vi "FilterWheelPan.vi"(8 "error in (no error)":errorcluster caption="entrée d'erreur (pas d'erreur)", 11 "AppliedMotionDrive.lvclass":refnum<class "AppliedMotionDrive.lvclass">) -> (0 "error out":errorcluster caption="sortie d'erreur", 3 "AppliedMotionDrive.lvclass Out":refnum<class "AppliedMotionDrive.lvclass">)   [LabVIEW 2019, in "AppliedMotionDrive.lvclass"]
uses:
  AppliedMotionDrive.lvclass
  C:/Programmes Labview/LabscanV1A/DevicesClass/BaseDevice/BaseDevice.lvclass
  AppliedMotionDrive.lvclass/AppliedMotionDrive.ctl
  BaseDevice/ClassQueueMess.ctl
  BaseDevice/Accessor/GetClassEvent.vi
panel:
  in  "Auto APD":bool
  out "ESP300Mirror":u16=1
  out "ESP300Filters":u16=1
  out "APDsRefs":refnum<vi>[](array[refnum])
  out "LampRefs":refnum<vi>[](array[refnum])
  out "DelayedClosed":bool caption="Confirm"
  out "Delay (hours)":dbl format="%#g"
  out "RéfMenu":refnum<k9>
  in  "White Lamp":bool
  in  "MainProgQEvent":refnum<user-event>
  in  "MainProgQ":refnum<queue>
  out "Offet(Units)":dbl caption="Offset(Units)"
  in  "APDs":bool
  in  "PosDelta(Units)":dbl caption="Pos delta(mm)"
  in  "Con":bool
  in  "TimeoutCnt":u32
  in  "Err":bool
  out "DisAtPos":bool
  out "Acq":bool
  in  "Filter pos(Units)":dbl caption="FiltPos(mm)"
  in  "Home":bool
  in  "En":bool
  in  "Filters":u16(ring) items=["test"]
  out "InstrName":string="Filter Wheel"
  out "Moving":bool
  in  "Stop Move":bool
  in  "Position(Units)":dbl caption="Position(mm)"
  in  "Stop":bool
  out "Init Program":bool
  # "this MUST labeled with class name"
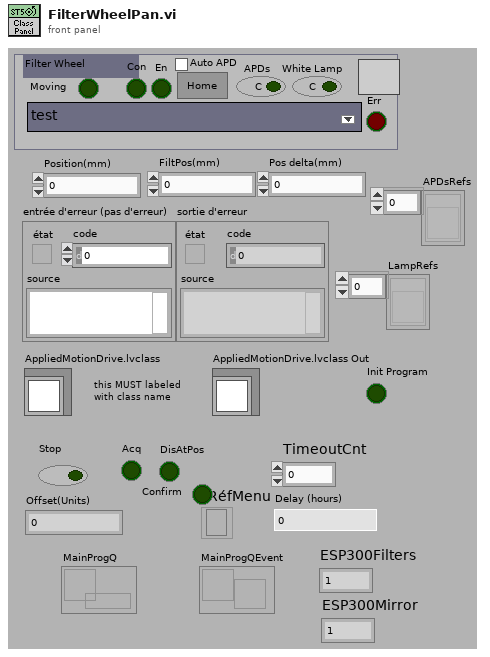
[diagram p1: front panel]
types:
  T1 = cluster{"Enabled":bool, "Sampling":bool, "Fault":bool, "In Position":bool, "Moving":bool, "Jogging":bool, "Stopping":bool, "Wait Input":bool, "Saving":bool, "Alarm":bool, "Homing":bool, "Waiting":bool, "Wait Time":bool, "Wizard":bool, "Checking Enc":bool, "Q mode":bool, "Initializing":bool}
  T2 = cluster{"Vitesse (Tour/s)":dbl, "Accél":dbl, "Décél":dbl, "Accél Max":dbl, "Idle Current (A) ":dbl}
  T3 = cluster{"Vitesse (Tour/s)":dbl, "Accél":dbl, "Décél":dbl}
  T4 = typedef "ClassQueueMess.ctl" = u16
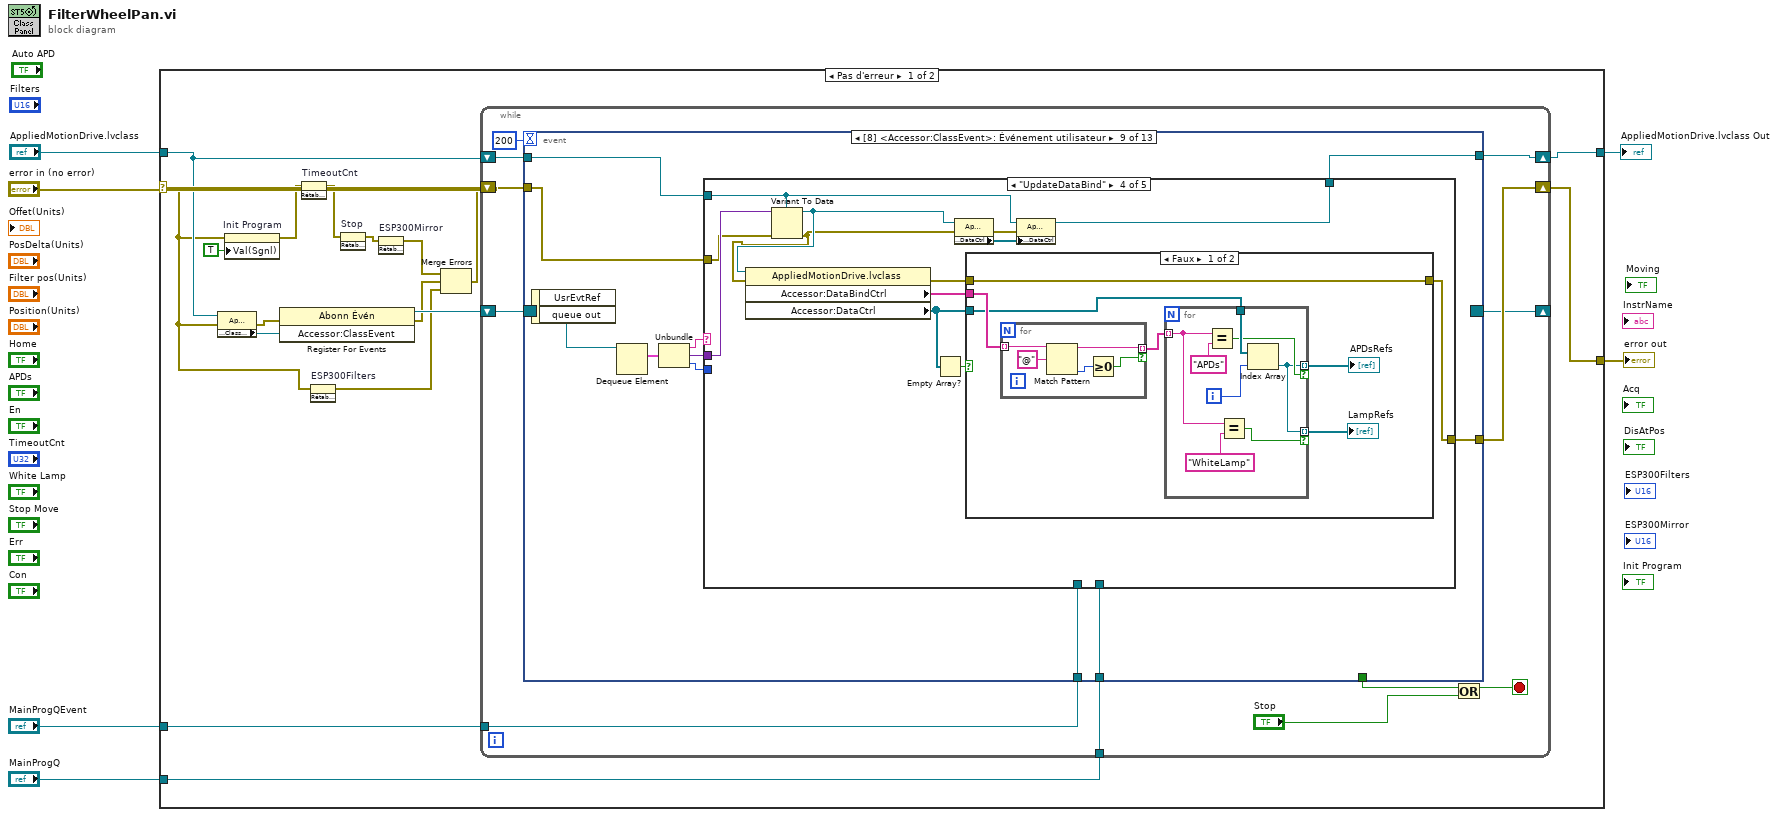
[diagram p0: block diagram]
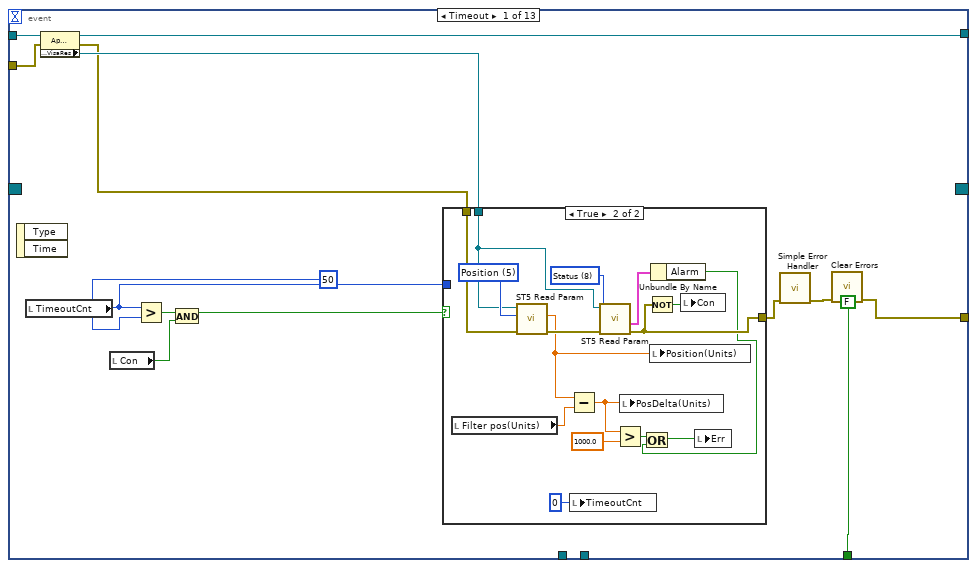
[diagram p2: hidden frame]
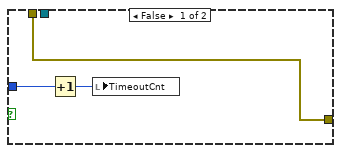
[diagram p3: hidden frame]
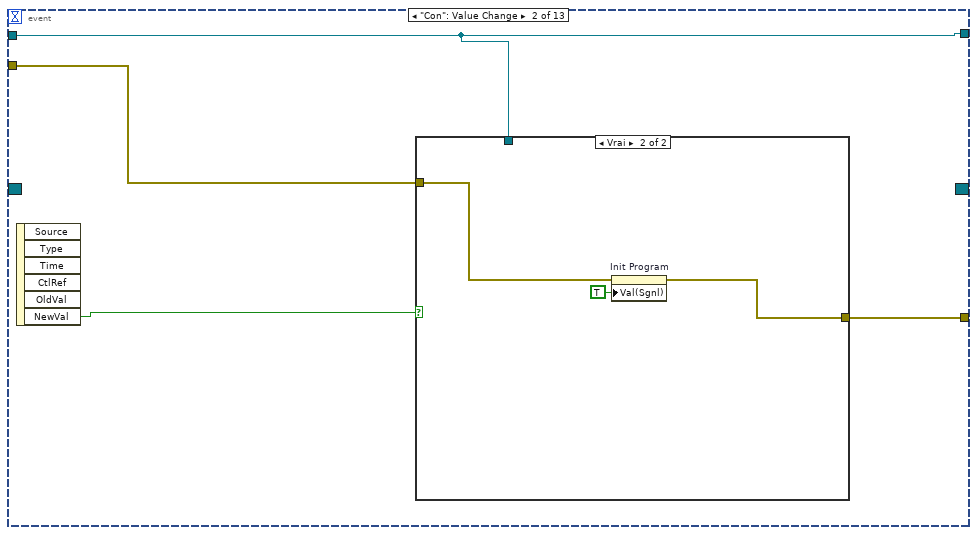
[diagram p4: hidden frame]
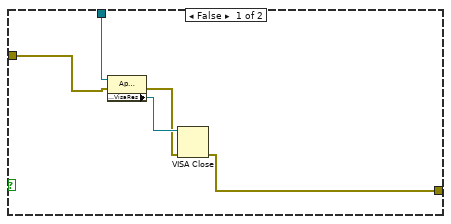
[diagram p5: hidden frame]
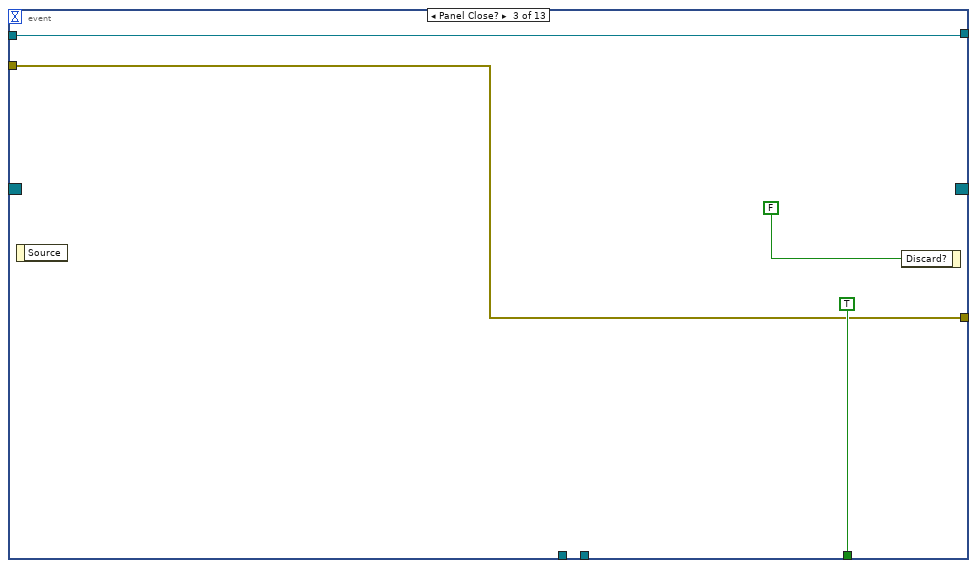
[diagram p6: hidden frame]
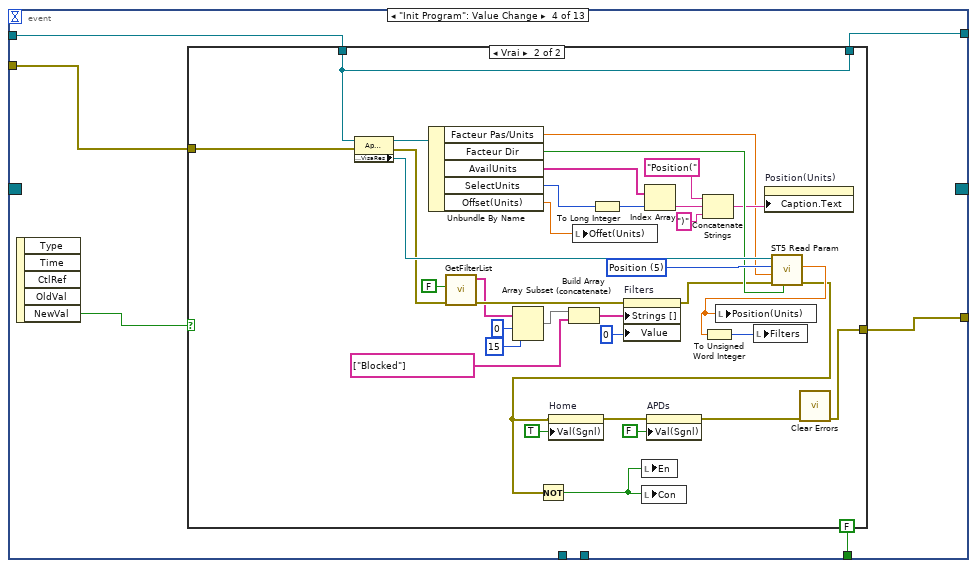
[diagram p7: hidden frame]
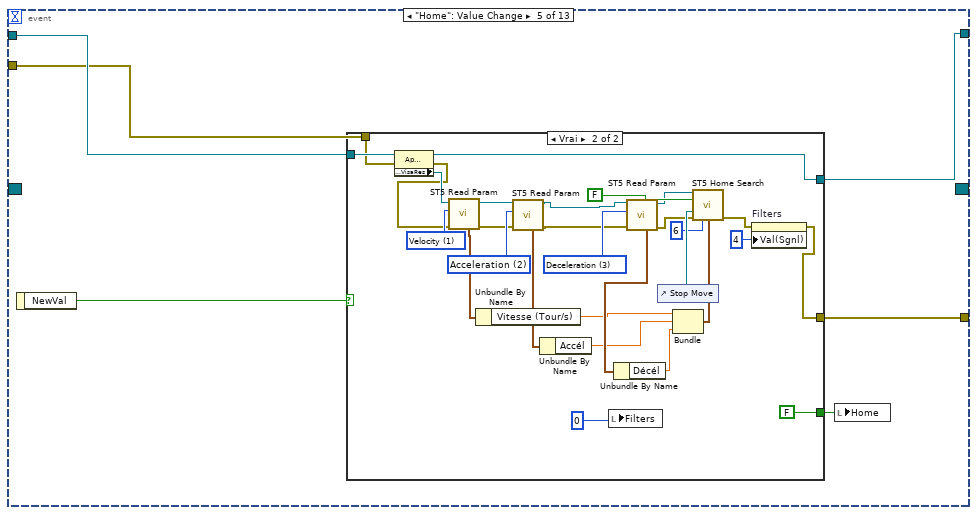
[diagram p9: hidden frame]
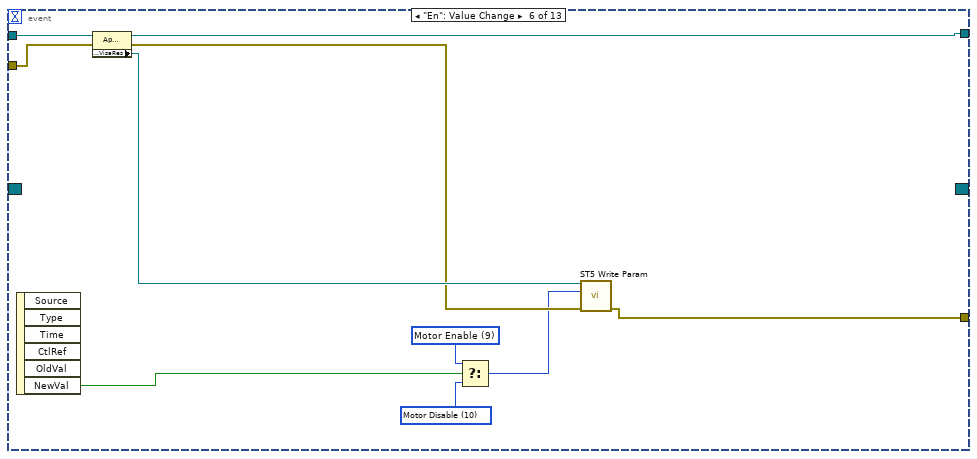
[diagram p11: hidden frame]
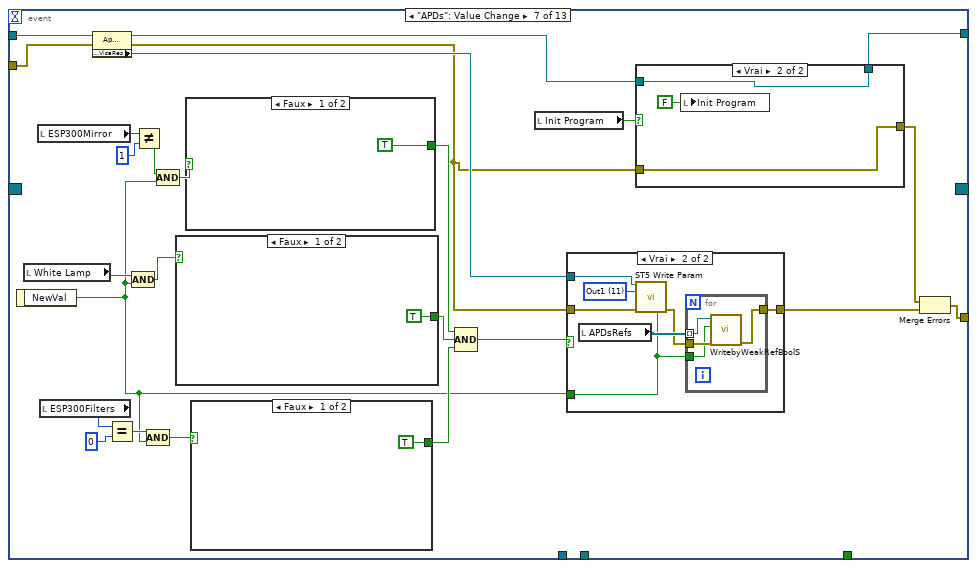
[diagram p12: hidden frame]
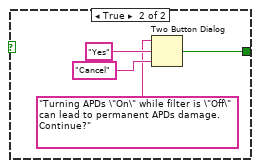
[diagram p14: hidden frame]
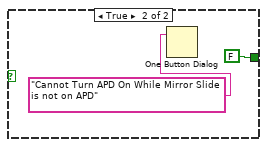
[diagram p15: hidden frame]
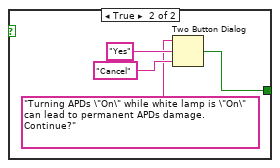
[diagram p16: hidden frame]
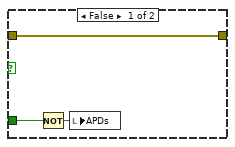
[diagram p17: hidden frame]
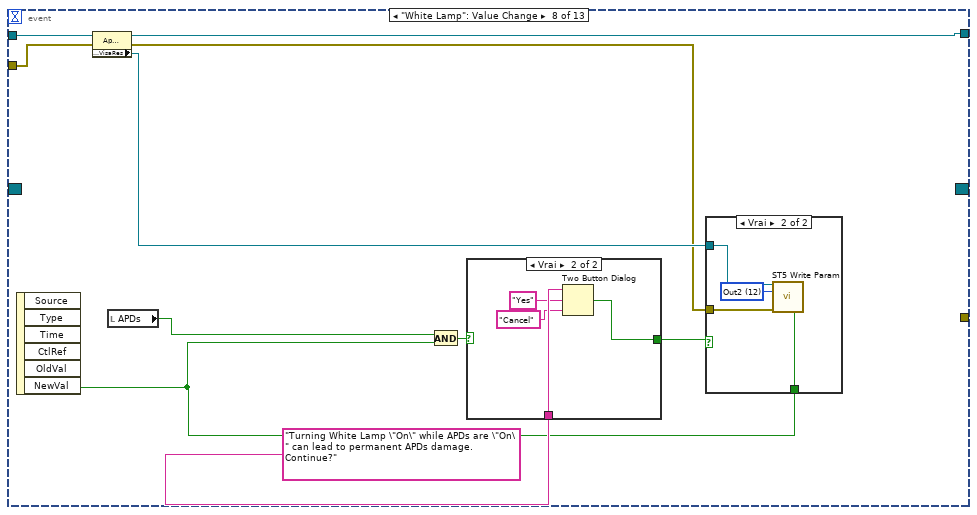
[diagram p18: hidden frame]
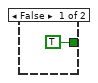
[diagram p19: hidden frame]
diagram:
  n1 = case shown="Pas d'erreur" "error in (no error)" {
    selector: "error in (no error)" -> [w8 w456]
    tunnel: [w23 w456] -> w5
    tunnel: "AppliedMotionDrive.lvclass" -> [w11 w455]
    tunnel: [w14 w455] -> w3
    tunnel: "MainProgQEvent" -> [w13 _]
    tunnel: "MainProgQ" -> [w12 _]
    frame No Error {
      n2 = property class="AppliedMotionDrive.lvclass"(reference=w11, error in=w8) -> (error out=w19:errorcluster, "Accessor:ClassEvent"=w20:refnum<user-event>)  [unwired: 1 out]
      n3 = property on="Init Program" class="Bool (strict)"(error in=w8, "Val(Sgnl)"=TRUE ("Valeur (Signalisation)")) -> (error out=w16:errorcluster)  [unwired: 1 in, 1 out]
      n4 = register-events(error in=w19, w20) -> (reference out=w21:refnum<event-registration>, error out=w18:errorcluster)  [unwired: 1 in]
      n5 = invoke on="TimeoutCnt" class="NumNb (strict)" method="RétablirValParDéfaut"(error in=w16) -> (error out=w15:errorcluster)  [unwired: 2 in, 2 out]
      n6 = invoke on="ESP300Filters" class="NumNb (strict)" method="RétablirValParDéfaut"(error in=w8) -> (error out=w7:errorcluster)  [unwired: 2 in, 2 out]
      n7 = invoke on="Stop" class="Bool (strict)" method="RétablirValParDéfaut"(error in=w15) -> (error out=w10:errorcluster)  [unwired: 2 in, 2 out]
      n8 = invoke on="ESP300Mirror" class="NumNb (strict)" method="RétablirValParDéfaut"(error in=w10) -> (error out=w9:errorcluster)  [unwired: 2 in, 2 out]
      n9 = Merge Errors(w9, w18, w7) -> (w17:errorcluster)
      n10 = while {
        shift-right: [w33] -> w23
        shift-left: w17 -> [w34]
        shift-right: [w26] -> w14
        shift-left: w11 -> [w27]
        shift-right: [w28] -> _
        shift-left: w21 -> [w29]
        tunnel: w13 -> [w25]
        tunnel: w12 -> [w24]
        stop <- w31 stop-if-true
        n11 = event shown="[8] <Accessor:ClassEvent>: Événement utilisateur" {
          selector: w29 -> [_ _ _ _ _ _ _ _ _ _ _ _ _]
          dyn-events: [_ _ _ _ _ _ _ _ _ _ _ _ _] -> w28
          timeout: 200 -> [_ _ _ _ _ _ _ _ _ _ _ _ _]
          tunnel: w34 -> [w42 w71 w82 w89 w129 w172 w198 w239 w262 w329 w395 w415 w453]
          tunnel: [w38 w70 w82 w88 w128 w166 w178 _ w254 w326 _ w414 w453] -> w33
          tunnel: [FALSE _ TRUE FALSE _ _ _ _ _ _ _ _ _] -> w32
          tunnel: w27 -> [w48 w69 w81 w86 w130 w175 w200 w242 w256 w323 w396 w416 w454]
          tunnel: [w44 w69 w81 w85 w131 w174 w180 w241 w255 w322 w397 w417 w454] -> w26
          tunnel: w25 -> [_ _ _ _ _ _ _ _ w253 _ _ _ _]
          tunnel: w24 -> [_ _ _ _ _ _ _ _ w252 _ _ _ _]
          event Timeout {
            n12 = event-data() -> ()  [unwired: 1 in, 2 out]
            n13 = local read "TimeoutCnt"() -> (w45:u32)
            n14 = property class="AppliedMotionDrive.lvclass"(reference=w48, error in=w42) -> (reference out=w44:refnum<class "AppliedMotionDrive.lvclass">, error out=w37:errorcluster, "Accessor:VisaRes"=w43:refnum<visa-resource-name>)
            n15 = local read "Con"() -> (w40:bool)
            n16 = Greater?(x=w45, y=u32 50) -> (0:w46:bool)
            n17 = And(x=w46, y=w40) -> (x .and. y?=w41:bool)
            n18 = case shown="Faux" w41 {
              tunnel: w45 -> [w52 _]
              tunnel: w37 -> [w50 w68]
              tunnel: [w50 w64] -> w36
              tunnel: w43 -> [_ w54]
              frame False {
                n19 = Increment(x=w52) -> (x+1=w51:u32)
                n20 = local write "TimeoutCnt"(w51) -> ()
              }
              frame True {
                w63 = u16 8 items=["All", "Velocity", "Acceleration", "Deceleration", "Max Acceleration", "Position", "Step/Rev", "Alarm Code", "Status", "Idle Current"] ("Parameters")
                w66 = u16 5 items=["All", "Velocity", "Acceleration", "Deceleration", "Max Acceleration", "Position", "Step/Rev", "Alarm Code", "Status", "Idle Current"] ("Parameters")
                n21 = local read "Filter pos(Units)"() -> (w60:dbl)
                n22 = call <userlib>:"ST5 Read Param.vi"("error in (no error)"=w68, "Parameters"=w66, "Port COM"=w54) -> ("error out"=w65:errorcluster, "Position"=w61:dbl)  [unwired: 2 in, 5 out]
                n23 = Subtract(x=w61, y=w60) -> (x-y=w59:dbl)
                n24 = local write "TimeoutCnt"(u32 0 ("TimeoutCnt")) -> ()
                n25 = call <userlib>:"ST5 Read Param.vi"("error in (no error)"=w65, "Parameters"=w63, "Port COM"=w54) -> ("error out"=w64:errorcluster, "Status"=w62:T1)  [unwired: 2 in, 5 out]
                n26 = Greater?(x=w59, y=1000.0) -> (0:w57:bool)
                n27 = local write "PosDelta(Units)"(w59) -> ()
                n28 = Not(x=w64) -> (.not. x?=w53:bool)
                n29 = local write "Position(Units)"(w61) -> ()
                n30 = Unbundle By Name(w62) -> ("Alarm"=w55:bool)
                n31 = Or(x=w57, y=w55) -> (x .or. y?=w56:bool)
                n32 = local write "Con"(w53) -> ()
                n33 = local write "Err"(w56) -> ()
              }
            }
            n34 = call <vilib>:"Simple Error Handler.vi"("error in (no error)"=w36) -> ("error out"=w39:errorcluster)  [unwired: 4 in, 4 out]
            n35 = call <vilib>:"Clear Errors.vi"("error in (no error)"=w39) -> ("error out"=w38:errorcluster)  [unwired: 5 in, 1 out]
          }
          event "Con": Value Change {
            n36 = event-data() -> ("NewVal"=w72:bool)  [unwired: 1 in, 5 out]
            n37 = case shown="Vrai" w72 {
              tunnel: w71 -> [w74 w79]
              tunnel: [w73 w78] -> w70
              tunnel: w69 -> [w75 _]
              frame False {
                n38 = property class="AppliedMotionDrive.lvclass"(reference=w75, error in=w74) -> (error out=w76:errorcluster, "Accessor:VisaRes"=w77:refnum<visa-resource-name>)  [unwired: 1 out]
                n39 = VISA Close(VISA resource name=w77, error in (no error)=w76) -> (error out=w73:errorcluster)
              }
              frame True {
                n40 = property on="Init Program" class="Bool (strict)"(error in=w79, "Val(Sgnl)"=TRUE ("Valeur (Signalisation)")) -> (error out=w78:errorcluster)  [unwired: 1 in, 1 out]
              }
            }
          }
          event Panel Close? {
            n41 = event-data() -> ()  [unwired: 1 in, 1 out]
            n42 = event-data("Discard?"=FALSE ("Rejeter ?")) -> ()  [unwired: 1 in, 1 out]
          }
          event "Init Program": Value Change {
            n43 = event-data() -> ("NewVal"=w90:bool)  [unwired: 1 in, 4 out]
            n44 = case shown="Vrai" w90 {
              tunnel: w89 -> [w92 w126]
              tunnel: [w92 w94] -> w88
              tunnel: w86 -> [w91 w95]
              tunnel: [w91 w95] -> w85
              frame False {
              }
              frame True {
                w127 = u16 5 items=["All", "Velocity", "Acceleration", "Deceleration", "Max Acceleration", "Position", "Step/Rev", "Alarm Code", "Status"] ("Parameters")
                n45 = property class="AppliedMotionDrive.lvclass"(reference=w95, error in=w126) -> (reference out=w125:refnum<class "AppliedMotionDrive.lvclass">, error out=w104:errorcluster, "Accessor:VisaRes"=w124:refnum<visa-resource-name>)
                n46 = Unbundle By Name(w125) -> ("Facteur Pas/Units"=w115:dbl, "Facteur Dir"=w123:bool, "AvailUnits"=w121:string[], "SelectUnits"=w120:u8, "Offset(Units)"=w98:dbl)
                n47 = call "GetFilterList.vi"("Error in"=w104, "Write"=FALSE) -> ("Error out"=w109:errorcluster, "Filter names out"=w106:string[])  [unwired: 4 in]
                n48 = Array Subset(array=w106, index=0 ("indice"), length=15 ("longueur")) -> (w100:string[])
                n49 = Build Array (concatenate)(w100, string[] ["Blocked"] ("tableau")) -> (w99:string[])
                n50 = local write "Offet(Units)"(w98) -> ()
                n51 = To Long Integer(number=w120) -> (32bit integer=w116:i32)
                n52 = property on="Filters" class="MDér (strict)"(error in=w109, "Strings []"=w99, "Value"=0) -> (error out=w103:errorcluster)  [unwired: 1 in, 1 out]
                n53 = Index Array(array=w121, index=w116) -> (element=w119:string)
                n54 = Concatenate Strings("Position(" ("chaîne"), w119, ")" ("expression régulière")) -> (w117:string)
                n55 = property on="Position(Units)" class="NumNb (strict)"("Caption.Text"=w117) -> ()  [unwired: 2 in, 2 out]
                n56 = call <userlib>:"ST5 Read Param.vi"("Facteur Dir"=w123, "error in (no error)"=w103, "Facteur Pas"=w115, "Parameters"=w127, "Port COM"=w124) -> ("error out"=w110:errorcluster, "Position"=w114:dbl)  [unwired: 5 out]
                n57 = Not(x=w110) -> (.not. x?=w112:bool)
                n58 = property on="Home" class="Bool (strict)"(error in=w110, "Val(Sgnl)"=TRUE ("Valeur (Signalisation)")) -> (error out=w111:errorcluster)  [unwired: 1 in, 1 out]
                n59 = local write "En"(w112) -> ()
                n60 = local write "Con"(w112) -> ()
                n61 = property on="APDs" class="Bool (strict)"(error in=w111, "Val(Sgnl)"=FALSE ("Valeur (Signalisation)")) -> (error out=w93:errorcluster)  [unwired: 1 in, 1 out]
                n62 = To Unsigned Word Integer(number=w114) -> (unsigned 16bit integer=w113:u16)
                n63 = local write "Position(Units)"(w114) -> ()
                n64 = local write "Filters"(w113) -> ()
                n65 = call <vilib>:"Clear Errors.vi"("error in (no error)"=w93) -> ("error out"=w94:errorcluster)  [unwired: 5 in, 1 out]
              }
            }
          }
          event "Home": Value Change {
            n66 = event-data() -> ("NewVal"=w133:bool)  [unwired: 1 in]
            n67 = case shown="Vrai" w133 {
              selector: w133 -> [w136 _]
              tunnel: [w136 FALSE ("Home")] -> w132
              tunnel: [w135 w163] -> w131
              tunnel: w130 -> [w135 w164]
              tunnel: w129 -> [w134 w162]
              tunnel: [w134 w137] -> w128
              frame False {
              }
              frame True {
                w149 = u16 3 items=["All", "Velocity", "Acceleration", "Deceleration", "Max Acceleration", "Position", "Step/Rev", "Alarm Code", "Status", "Idle Current"] ("Parameters")
                w156 = u16 2 items=["All", "Velocity", "Acceleration", "Deceleration", "Max Acceleration", "Position", "Step/Rev", "Alarm Code", "Status", "Idle Current"] ("Parameters")
                w157 = u16 1 items=["All", "Velocity", "Acceleration", "Deceleration", "Max Acceleration", "Position", "Step/Rev", "Alarm Code", "Status", "Idle Current"] ("Parameters")
                n68 = property class="AppliedMotionDrive.lvclass"(reference=w164, error in=w162) -> (reference out=w163:refnum<class "AppliedMotionDrive.lvclass">, error out=w153:errorcluster, "Accessor:VisaRes"=w158:refnum<visa-resource-name>)
                n69 = call <userlib>:"ST5 Read Param.vi"("error in (no error)"=w153, "Parameters"=w157, "Port COM"=w158) -> ("error out"=w154:errorcluster, "Port COM Out"=w155:refnum<visa-resource-name>, "Speed Par"=w152:T2)  [unwired: 2 in, 4 out]
                n70 = Unbundle By Name(w152) -> ("Vitesse (Tour/s)"=w143:dbl)
                n71 = call <userlib>:"ST5 Read Param.vi"("error in (no error)"=w154, "Parameters"=w156, "Port COM"=w155) -> ("error out"=w147:errorcluster, "Port COM Out"=w148:refnum<visa-resource-name>, "Speed Par"=w151:T2)  [unwired: 2 in, 4 out]
                n72 = Unbundle By Name(w151) -> ("Accél"=w142:dbl)
                n73 = local write "Filters"(u16 0) -> ()
                n74 = call <userlib>:"ST5 Read Param.vi"("error in (no error)"=w147, "Parameters"=w149, "Port COM"=w148) -> ("error out"=w146:errorcluster, "Port COM Out"=w145:refnum<visa-resource-name>, "Speed Par"=w150:T2)  [unwired: 2 in, 4 out]
                n75 = Unbundle By Name(w150) -> ("Décél"=w141:dbl)
                n76 = control-ref of="Stop Move"() -> (w160:refnum<vi>)
                n77 = Bundle("Vitesse (Tour/s)"=w143, "Accél"=w142, "Décél"=w141) -> (w144:T3)  [unwired: 1 in]
                n78 = call <userlib>:"ST5 Home Search.vi"("Port COM"=w145, "Home Dir"=FALSE, "Ext Stop Ref"=w160, "error in (no error)"=w146, "HomeInput"=u8 6, "Normal Speed Par"=w144) -> ("error out"=w138:errorcluster)  [unwired: 5 in, 4 out]
                n79 = property on="Filters" class="MDér (strict)"(error in=w138, "Val(Sgnl)"=u16 4 ("Valeur (Signalisation)")) -> (error out=w137:errorcluster)  [unwired: 1 in, 1 out]
              }
            }
            n80 = local write "Home"(w132) -> ()
          }
          event "En": Value Change {
            w168 = u16 10 items=["Velocity", "Acceleration", "Deceleration", "Max Acceleration", "Zero", "Save", "Encoder Res", "Clear Alarm", "Home Search", "Motor Enable", "Motor Disable"] ("Parameters")
            w169 = u16 9 items=["Velocity", "Acceleration", "Deceleration", "Max Acceleration", "Zero", "Save", "Encoder Res", "Clear Alarm", "Home Search", "Motor Enable", "Motor Disable"] ("Parameters")
            n81 = event-data() -> ("NewVal"=w170:bool)  [unwired: 1 in, 5 out]
            n82 = property class="AppliedMotionDrive.lvclass"(reference=w175, error in=w172) -> (reference out=w174:refnum<class "AppliedMotionDrive.lvclass">, error out=w171:errorcluster, "Accessor:VisaRes"=w173:refnum<visa-resource-name>)
            n83 = Select(t=w169, s=w170, f=w168) -> (s? t:f=w167:u16)
            n84 = call <userlib>:"ST5 Write Param.vi"("Port COM"=w173, "Parameters"=w167, "error in (no error)"=w171) -> ("error out"=w166:errorcluster)  [unwired: 11 in, 1 out]
          }
          event "APDs": Value Change {
            n85 = event-data() -> ("NewVal"=w183:bool)  [unwired: 1 in]
            n86 = local read "White Lamp"() -> (w196:bool)
            n87 = local read "ESP300Mirror"() -> (w193:u16)
            n88 = local read "ESP300Filters"() -> (w188:u16)
            n89 = property class="AppliedMotionDrive.lvclass"(reference=w200, error in=w198) -> (reference out=w181:refnum<class "AppliedMotionDrive.lvclass">, error out=w179:errorcluster, "Accessor:VisaRes"=w199:refnum<visa-resource-name>)
            n90 = Equal?(x=w188, y=u16 0) -> (x = y?=w184:bool)
            n91 = Compound Arithmetic op=AND ("Opérateur arithmétique")(w196, w183) -> (w195:bool)
            n92 = Not Equal?(x=w193, y=u16 1) -> (x != y?=w186:bool)
            n93 = Compound Arithmetic op=AND ("Opérateur arithmétique")(w184, w183) -> (w182:bool)
            n94 = Compound Arithmetic op=AND ("Opérateur arithmétique")(w186, w183) -> (w185:bool)
            n95 = case shown="Faux" w195 {
              tunnel: [TRUE w216] -> w197
              frame False {
              }
              frame True {
                n96 = Two Button Dialog(message="Turning APDs \"On\" while white lamp is \"On\" can lead to permanent APDs damage. Continue?", 1:"Cancel" ("Nom du bouton F (\"Annuler\")"), 2:"Yes" ("Nom du bouton V (\"OK\")")) -> (T button?=w216:bool)
              }
            }
            n97 = case shown="Faux" w185 {
              tunnel: [TRUE FALSE] -> w190
              frame False {
              }
              frame True {
                n98 = One Button Dialog(message="Cannot Turn APD On While Mirror Slide is not on APD") -> ()  [unwired: 1 in, 1 out]
              }
            }
            n99 = case shown="Faux" w182 {
              tunnel: [TRUE w208] -> w187
              frame False {
              }
              frame True {
                n100 = Two Button Dialog(message="Turning APDs \"On\" while filter is \"Off\" can lead to permanent APDs damage. Continue?", 1:"Cancel" ("Nom du bouton F (\"Annuler\")"), 2:"Yes" ("Nom du bouton V (\"OK\")")) -> (T button?=w208:bool)
              }
            }
            n101 = Compound Arithmetic op=AND ("Opérateur arithmétique")(w190, w197, w187) -> (w191:bool)
            n102 = local read "Init Program"() -> (w176:bool)
            n103 = case shown="Vrai" w191 {
              tunnel: w199 -> [_ w228]
              tunnel: w179 -> [w221 w227]
              tunnel: w183 -> [w220 w222]
              tunnel: [w221 w223] -> w194
              frame False {
                n104 = Not(x=w220) -> (.not. x?=w219:bool)
                n105 = local write "APDs"(w219) -> ()
              }
              frame True {
                w226 = u16 11 items=["Velocity", "Acceleration", "Deceleration", "Max Acceleration", "Zero", "Save", "Encoder Res", "Clear Alarm", "Home Search", "Motor Enable", "Motor Disable", "Out1", "Out2", "Out3", "Out4"] ("Parameters")
                n106 = local read "APDsRefs"() -> (w225:refnum<vi>[])
                n107 = call <userlib>:"ST5 Write Param.vi"("Port COM"=w228, "Parameters"=w226, "error in (no error)"=w227, "Output Active"=w222) -> ("error out"=w224:errorcluster)  [unwired: 10 in, 1 out]
                n108 = for {
                  tunnel: w225 -> [w232] mode=indexing
                  tunnel: w224 -> [w231]
                  tunnel: [w230] -> w223
                  tunnel: w222 -> [w229]
                  n109 = call <userlib>:"WritebyWeakRefBoolS.vi"("error in"=w231, "Valeur"=w229, "Control Ref"=w232) -> ("error out"=w230:errorcluster)  [unwired: 8 in]
                }
              }
            }
            n110 = case shown="Vrai" w176 {
              tunnel: w181 -> [w202 w204]
              tunnel: [w202 w204] -> w180
              tunnel: w179 -> [w201 w203]
              tunnel: [w201 w203] -> w177
              frame False {
              }
              frame True {
                n111 = local write "Init Program"(FALSE ("Init Program")) -> ()
              }
            }
            n112 = Merge Errors(w177, w194) -> (w178:errorcluster)
          }
          event "White Lamp": Value Change {
            n113 = event-data() -> ("NewVal"=w233:bool)  [unwired: 1 in, 5 out]
            n114 = property class="AppliedMotionDrive.lvclass"(reference=w242, error in=w239) -> (reference out=w241:refnum<class "AppliedMotionDrive.lvclass">, error out=w238:errorcluster, "Accessor:VisaRes"=w240:refnum<visa-resource-name>)
            n115 = local read "APDs"() -> (w235:bool)
            n116 = And(x=w235, y=w233) -> (x .and. y?=w234:bool)
            n117 = case shown="Vrai" w234 {
              tunnel: [TRUE w244] -> w237
              tunnel: "Turning White Lamp \"On\" while APDs are \"On\" can lead to permanent APDs damage. Continue?" ("message") -> [_ w247]
              frame False {
              }
              frame True {
                n118 = Two Button Dialog(message=w247, 1:"Cancel" ("Nom du bouton F (\"Annuler\")"), 2:"Yes" ("Nom du bouton V (\"OK\")")) -> (T button?=w244:bool)
              }
            }
            n119 = case shown="Vrai" w237 {
              tunnel: w240 -> [_ w251]
              tunnel: w238 -> [_ w250]
              tunnel: w233 -> [_ w248]
              frame False {
              }
              frame True {
                w249 = u16 12 items=["Velocity", "Acceleration", "Deceleration", "Max Acceleration", "Zero", "Save", "Encoder Res", "Clear Alarm", "Home Search", "Motor Enable", "Motor Disable", "Out1", "Out2", "Out3", "Out4"] ("Parameters")
                n120 = call <userlib>:"ST5 Write Param.vi"("Port COM"=w251, "Parameters"=w249, "error in (no error)"=w250, "Output Active"=w248) -> ()  [unwired: 10 in, 2 out]
              }
            }
          }
          event User Event {
            n121 = event-data() -> ("queue out"=w261:refnum<queue>)  [unwired: 1 in, 1 out]
            n122 = Dequeue Element(queue=w261) -> (element=w260:cluster{"Message":string, "Data":variant, i32})  [unwired: 2 in, 3 out]
            n123 = Unbundle(w260) -> ("Message"=w259:string, "Data"=w257:variant, w258:i32)
            n124 = case shown="\"UpdateDataBind\"" w259 {
              tunnel: w262 -> [w263 w266 w271 w276 w311]
              tunnel: w257 -> [_ _ w274 w282 _]
              tunnel: w258 -> [_ _ _ _ _]
              tunnel: w256 -> [w264 w267 w273 w278 w312]
              tunnel: [w264 w267 w272 w277 w312] -> w255
              tunnel: [w263 w265 w270 w283 w310] -> w254
              tunnel: w253 -> [_ _ _ _ w309]
              tunnel: w252 -> [_ _ _ _ w308]
              frame Default {
              }
              frame "ShowDiag" {
                n125 = control-ref of="ce VI"() -> (w268:refnum<vi>)
                n126 = call <userlib>:"AnimExecGen.vi"("ErrorIn(No Error)"=w266, "Animer l'exécution ?"=TRUE, "ViRef"=w268) -> ("sortie d'erreur"=w265:errorcluster)  [unwired: 8 in]
              }
              frame "UpdateClassData" {
                n127 = Variant To Data(error in=w271, type=w273, Variant=w274) -> (data=w272:refnum<class "AppliedMotionDrive.lvclass">, error out=w270:errorcluster)
              }
              frame "UpdateDataBind" {
                n128 = Variant To Data(error in=w276, type=w278, Variant=w282) -> (data=w279:refnum<class "AppliedMotionDrive.lvclass">, error out=w275:errorcluster)
                n129 = property class="AppliedMotionDrive.lvclass"(reference=w279, error in=w275) -> (error out=w285:errorcluster, "Accessor:DataBindCtrl"=w287:string[], "Accessor:DataCtrl"=w286:refnum<vi>[])  [unwired: 1 out]
                n130 = Empty Array?(array=w286) -> (empty?=w284:bool)
                n131 = property class="AppliedMotionDrive.lvclass"(reference=w279, error in=w275) -> (error out=w281:errorcluster, "Accessor:DataCtrl"=w280:refnum<vi>[])  [unwired: 1 out]
                n132 = case shown="Faux" w284 {
                  tunnel: w287 -> [w292 _]
                  tunnel: w286 -> [w290 _]
                  tunnel: w285 -> [w293 w307]
                  tunnel: [w293 w307] -> w283
                  frame False {
                    n133 = for {
                      tunnel: w292 -> [w306] mode=indexing
                      tunnel: [w304] -> w291 mode=indexing if=w303
                      n134 = Match Pattern(string=w306, regular expression="@" ("expression régulière")) -> (before substring=w304:string, offset past match=w302:i32)  [unwired: 1 in, 2 out]
                      n135 = Greater Or Equal To 0?(x=w302) -> (x >= 0?=w303:bool)
                    }
                    n136 = for {
                      tunnel: w291 -> [w297] mode=indexing
                      tunnel: w290 -> [w300]
                      tunnel: [w295] -> w289 mode=indexing if=w298
                      tunnel: [w295] -> w288 mode=indexing if=w294
                      i -> [w299]
                      n137 = Equal?(x=w297, y="APDs" ("nom (aucun)")) -> (x = y?=w298:bool)
                      n138 = Equal?(x=w297, y="WhiteLamp" ("nom (aucun)")) -> (x = y?=w294:bool)
                      n139 = Index Array(array=w300, index=w299) -> (element=w295:refnum<vi>)
                    }
                    "APDsRefs" <- w289
                    "LampRefs" <- w288
                  }
                  frame True {
                  }
                }
                n140 = property class="AppliedMotionDrive.lvclass"(reference=w278, error in=w281, "Accessor:DataCtrl"=w280) -> (reference out=w277:refnum<class "AppliedMotionDrive.lvclass">)  [unwired: 1 out]
              }
              frame "UpdateMainClass" {
                n141 = Bundle By Name(cluster=cluster{"Message":string, "Data":variant, i32} {"Message"="", "Data"=variant, 0} ("élément"), "Data"=w312) -> (w313:cluster{"Message":string, "Data":variant, i32})
                n142 = Enqueue Element(queue=w308, element=w313, error in (no error)=w311) -> (queue out=w316:refnum<queue>, error out=w315:errorcluster)  [unwired: 1 in, 1 out]
                n143 = Generate User Event(user event=w309, event data cluster=w316, error in=w315) -> (error out=w310:errorcluster)  [unwired: 1 in, 1 out]
              }
            }
          }
          event "Filters": Value Change {
            n144 = event-data() -> ("OldVal"=w320:u16, "NewVal"=w321:u16)  [unwired: 1 in]
            n145 = local read "APDs"() -> (w317:bool)
            n146 = local read "Auto APD"() -> (w318:bool)
            n147 = property class="AppliedMotionDrive.lvclass"(reference=w323, error in=w329) -> (reference out=w322:refnum<class "AppliedMotionDrive.lvclass">, error out=w328:errorcluster, "Accessor:VisaRes"=w327:refnum<visa-resource-name>)
            n148 = Compound Arithmetic op=OR ("Opérateur arithmétique")(invert w317, w318) -> (w319:bool)
            n149 = Unbundle By Name(w322) -> ("Facteur Pas/Units"=w325:dbl, "Facteur Dir"=w324:bool)
            n150 = case shown="Vrai" w319 {
              tunnel: w328 -> [w331 w340]
              tunnel: w327 -> [_ w341]
              tunnel: [w331 w333] -> w326
              tunnel: w325 -> [_ w348]
              tunnel: w324 -> [_ w347]
              tunnel: w321 -> [_ w343]
              tunnel: w320 -> [w332 _]
              tunnel: w318 -> [_ _]
              tunnel: w317 -> [_ w342]
              frame False {
                n151 = local write "Filters"(w332) -> ()
                n152 = One Button Dialog(message="Modifying filters while APDs are On can be hazardous! Please close APDs first") -> ()  [unwired: 1 in, 1 out]
              }
              frame True {
                n153 = case shown="Faux" w342 {
                  selector: w342 -> [w359 w362]
                  tunnel: w341 -> [w360 w370]
                  tunnel: w340 -> [w361 w369]
                  tunnel: [w361 w365] -> w338
                  tunnel: [w360 w363] -> w339
                  tunnel: [w359 w362] -> w334
                  frame False {
                  }
                  frame True {
                    w364 = FALSE
                    w368 = u16 11 items=["Velocity", "Acceleration", "Deceleration", "Max Acceleration", "Zero", "Save", "Encoder Res", "Clear Alarm", "Home Search", "Motor Enable", "Motor Disable", "Out1", "Out2", "Out3", "Out4"] ("Parameters")
                    n154 = local read "APDsRefs"() -> (w367:refnum<vi>[])
                    n155 = call <userlib>:"ST5 Write Param.vi"("Port COM"=w370, "Parameters"=w368, "error in (no error)"=w369, "Output Active"=w364) -> ("Port COM Out"=w363:refnum<visa-resource-name>, "error out"=w366:errorcluster)  [unwired: 10 in]
                    n156 = call <userlib>:"WritebyWeakRefBoolArrS.vi"("error in"=w366, "Valeur"=w364, "Control Ref"=w367) -> ("error out"=w365:errorcluster)  [unwired: 8 in]
                  }
                }
                n157 = local read "Offet(Units)"() -> (w344:dbl)
                n158 = local write "Filters"(w343) -> ()
                n159 = To Double Precision Float(number=w343) -> (double precision float=w346:dbl)
                n160 = Add(x=w346, y=w344) -> (x+y=w345:dbl)
                n161 = case shown="0, Par défaut" w343 {
                  tunnel: w338 -> [w381 w391]
                  tunnel: w339 -> [w380 w390]
                  tunnel: [w379 w387] -> w335
                  tunnel: w348 -> [w378 w389]
                  tunnel: w347 -> [w377 w388]
                  tunnel: w345 -> [w373 _]
                  tunnel: w344 -> [_ w384]
                  tunnel: [w372 w383] -> w337
                  tunnel: [w371 w382] -> w336
                  frame 0, Default {
                    n162 = control-ref of="Stop Move"() -> (w376:refnum<vi>)
                    n163 = control-ref of="Position(Units)"() -> (w375:refnum<vi>)
                    n164 = call <userlib>:"ST5 Goto.vi"("Port COM"=w380, "Facteur Pas"=w378, "Facteur Dir"=w377, "Position"=w373, "PositionRef"=w375, "Ext Stop Ref"=w376, "error in (no error)"=w381, "Tolerance(units"=0.2) -> ("Port Out"=w371:refnum<visa-resource-name>, "Position Out"=w372:dbl, "error out"=w379:errorcluster)  [unwired: 1 in, 4 out]
                  }
                  frame 15 {
                    # "Blocked position"
                    n165 = control-ref of="Position(Units)"() -> (w393:refnum<vi>)
                    n166 = control-ref of="Stop Move"() -> (w394:refnum<vi>)
                    n167 = Add(x=w384, y=3.5 ("nombre")) -> (x+y=w385:dbl)
                    n168 = call <userlib>:"ST5 Goto.vi"("Port COM"=w390, "Facteur Pas"=w389, "Facteur Dir"=w388, "Position"=w385, "PositionRef"=w393, "Ext Stop Ref"=w394, "error in (no error)"=w391, "Tolerance(units"=0.2) -> ("Port Out"=w382:refnum<visa-resource-name>, "Position Out"=w383:dbl, "error out"=w387:errorcluster)  [unwired: 1 in, 4 out]
                  }
                }
                n169 = case shown="Faux" w334 {
                  tunnel: w336 -> [w349 w358]
                  tunnel: w335 -> [w350 w357]
                  tunnel: [w350 w353] -> w333
                  tunnel: [w349 w351] -> _
                  frame False {
                  }
                  frame True {
                    w352 = TRUE
                    w356 = u16 11 items=["Velocity", "Acceleration", "Deceleration", "Max Acceleration", "Zero", "Save", "Encoder Res", "Clear Alarm", "Home Search", "Motor Enable", "Motor Disable", "Out1", "Out2", "Out3", "Out4"] ("Parameters")
                    n170 = local read "APDsRefs"() -> (w355:refnum<vi>[])
                    n171 = call <userlib>:"ST5 Write Param.vi"("Port COM"=w358, "Parameters"=w356, "error in (no error)"=w357, "Output Active"=w352) -> ("Port COM Out"=w351:refnum<visa-resource-name>, "error out"=w354:errorcluster)  [unwired: 10 in]
                    n172 = call <userlib>:"WritebyWeakRefBoolArrS.vi"("error in"=w354, "Valeur"=w352, "Control Ref"=w355) -> ("error out"=w353:errorcluster)  [unwired: 8 in]
                  }
                }
                n173 = local write "Filter pos(Units)"(w337) -> ()
                n174 = local write "Position(Units)"(w337) -> ()
              }
            }
          }
          event "Filters": Shortcut Menu Selection (User) {
            n175 = event-data() -> ("ItemTag"=w398:string)  [unwired: 1 in, 7 out]
            n176 = case shown="\"Set Offset\"" w398 {
              tunnel: [w399 w404] -> w397
              tunnel: w396 -> [w399 w405]
              tunnel: w395 -> [_ w403]
              frame Default {
              }
              frame "Set Offset" {
                n177 = call "Boîte de dialogue utilisateur"("error in (no error)"=w403) -> ("Offset"=w400:dbl, "Save"=w401:bool, "error out"=w402:errorcluster)  [unwired: 16 in]
                n178 = case shown="Vrai" w401 {
                  tunnel: w405 -> [w406 w412]
                  tunnel: [w406 w411] -> w404
                  tunnel: w402 -> [_ w409]
                  tunnel: w400 -> [_ w407]
                  frame False {
                  }
                  frame True {
                    w410 = T4 1 items=["UpdateClassData", "UpdateMainClass", "UpdateDataBind", "ReInitDevice", "Custom", "ClosePan"] ("Menu déroulant")
                    n179 = Bundle By Name(cluster=w412, "Offset(Units)"=w407) -> (w408:refnum<class "AppliedMotionDrive.lvclass">)
                    n180 = local write "Offet(Units)"(w407) -> ()
                    n181 = call-dynamic "SetClassQueueMessage.vi"("ErrorIn(No Error)"=w409, "Menu déroulant"=w410, "AppliedMotionDrive.lvclass"=w408) -> ("AppliedMotionDrive.lvclass Out"=w411:refnum<class "AppliedMotionDrive.lvclass">)  [unwired: 7 in, 1 out]
                  }
                }
              }
            }
          }
          event "APDs": Shortcut Menu Selection (User) {
            n182 = event-data() -> ("CtlRef"=w413:refnum<vi>, "ItemTag"=w418:string)  [unwired: 1 in, 6 out]
            n183 = case shown="\"CloseAfterScan\"" w418 {
              selector: w418 -> [_ w422 w439]
              tunnel: [w420 w431 w443] -> w417
              tunnel: w416 -> [w420 w427 w443]
              tunnel: w415 -> [w419 w429 w441]
              tunnel: [w419 w430 w440] -> w414
              tunnel: w413 -> [_ _ _]
              frame Default {
              }
              frame "CloseAfterScan" {
                w424 = T4 1 items=["UpdateClassData", "UpdateMainClass", "UpdateDataBind", "ReInitDevice", "Custom", "ClosePan"] ("Menu déroulant")
                n184 = Unbundle By Name(w427) -> ("CloseAPD"=w426:bool)
                n185 = local read "RéfMenu"() -> (w425:refnum<k9>)
                n186 = Not(x=w426) -> (.not. x?=w421:bool)
                n187 = Set Menu Item Info(6:w421, 7:w422, 8:w429, 11:w425) -> (0:w428:errorcluster)  [unwired: 3 in, 1 out]
                n188 = Bundle By Name(cluster=w427, "CloseAPD"=w421) -> (w423:refnum<class "AppliedMotionDrive.lvclass">)
                n189 = call-dynamic "SetClassQueueMessage.vi"("ErrorIn(No Error)"=w428, "Menu déroulant"=w424, "AppliedMotionDrive.lvclass"=w423) -> ("sortie d'erreur"=w430:errorcluster, "AppliedMotionDrive.lvclass Out"=w431:refnum<class "AppliedMotionDrive.lvclass">)  [unwired: 7 in]
              }
              frame "DelayedClose" {
                n190 = local read "DelayedClosed"() -> (w435:bool)
                n191 = local read "RéfMenu"() -> (w442:refnum<k9>)
                n192 = local read "Delay (hours)"() -> (w438:dbl)
                n193 = case shown="Vrai" w435 {
                  tunnel: [w444 w446] -> w436
                  frame False {
                    n194 = call "Delayed close"() -> ("Delay (hours)"=→"Delay (hours)":dbl, "Confirm"=w444:bool)  [unwired: 17 in, 1 out]
                    "DelayedClosed" <- w444
                  }
                  frame True {
                    n195 = Two Button Dialog(message="Cancel Delayed Close?", 1:"No" ("Nom du bouton F (\"Annuler\")"), 2:"Yes" ("Nom du bouton V (\"OK\")")) -> (T button?=w447:bool)
                    n196 = Not(x=w447) -> (.not. x?=w446:bool)
                  }
                }
                n197 = Format Into String(format string="Time Left: %t" ("chaîne de format"), w438) -> (resulting string=w434:string)  [unwired: 2 in, 1 out]
                n198 = Select(t=w434, s=w435, f="" ("cas faux")) -> (s? t:f=w433:string)
                n199 = Set Menu Item Info(7:w439, 8:w441, 9:w436, 10:w433, 11:w442) -> (0:w440:errorcluster)  [unwired: 2 in, 1 out]
              }
            }
          }
          event "APDs": Shortcut Menu Activation? {
            n200 = event-data() -> ("MenuRef"=→"RéfMenu":refnum<k9>)  [unwired: 1 in, 6 out]
            n201 = event-data("Discard?"=FALSE ("Rejeter ?")) -> ()  [unwired: 1 in, 1 out]
          }
        }
        n202 = Or(x=w32, y="Stop") -> (x .or. y?=w31:bool)
      }
    }
    frame Error {
    }
  }
  "error out" <- w5
  "AppliedMotionDrive.lvclass Out" <- w3
